vi "Unit Test Array of Classes.vi"() -> ()   [LabVIEW 2019, in "Sports Unit Tests.lvclass"]
uses:
  Sports Unit Tests.lvclass
  Classes/Shaquille ONeal/Shaquille O'Neal.lvclass
  C:/DSCE code/Serialization/blueserializationdemo/Test/Sports/Classes/Human/Human.lvclass
  C:/DSCE code/Serialization/blueserializationdemo/Test/Sports/Classes/Sports Player/Sports Player.lvclass
  Classes/Adam Sandler/Adam Sandler.lvclass
  C:/DSCE code/Serialization/blueserializationdemo/Test/Sports/Classes/Golf Player/Golf Player.lvclass
  Classes/Human/Human.lvclass/Human.ctl
  Classes/Sports Player/Sports Player.lvclass/Sports Player.ctl
  Classes/Golf Player/Golf Player.lvclass/Golf Player.ctl
  Classes/Adam Sandler/Adam Sandler.lvclass/Adam Sandler.ctl
  Classes/Shaquille ONeal/Shaquille O'Neal.lvclass/Shaquille O'Neal.ctl
  Classes/Sports Player/Sports Player.lvclass
  Classes/Human/Write Age (years).vi
  Classes/Human/Write alive_.vi
  Classes/Human/Write Height (ft).vi
  Classes/Human/Write Name.vi
  Classes/Sports Player/Write Earnings (dollars).vi
  Classes/Sports Player/Write Professional_.vi
  Classes/Sports Player/Write Sponsor.vi
  Classes/Golf Player/Write # holes in one.vi
  Classes/Golf Player/Write League.vi
  Classes/Golf Player/Write longest drive (ft).vi
  Classes/Adam Sandler/Write Movie Name.vi
  Classes/Adam Sandler/Write Private number.vi
  Classes/Adam Sandler/Write Secret phrase.vi
  Classes/Shaquille ONeal/Write #slam dunks.vi
  Classes/Shaquille ONeal/Write Nickname.vi
  <vilib>/Utility/error.llb/Clear Errors.vi
  <vilib>/addons/_JKI Toolkits/Caraya/classes/Test/Define Test.vi
  <vilib>/addons/_JKI Toolkits/Caraya/classes/Assert/Assert Equal Value_Variant.vi
  <vilib>/addons/_JKI Toolkits/Caraya/classes/Assert/Assert Not Error.vi
  <vilib>/addons/_JKI Toolkits/Caraya/classes/Assert/Assert.lvclass
  <userlib>/Blue Origin/BlueSerialization/BlueSerializer/BlueSerializer.lvclass
panel:
  out "Table":string[][](table)
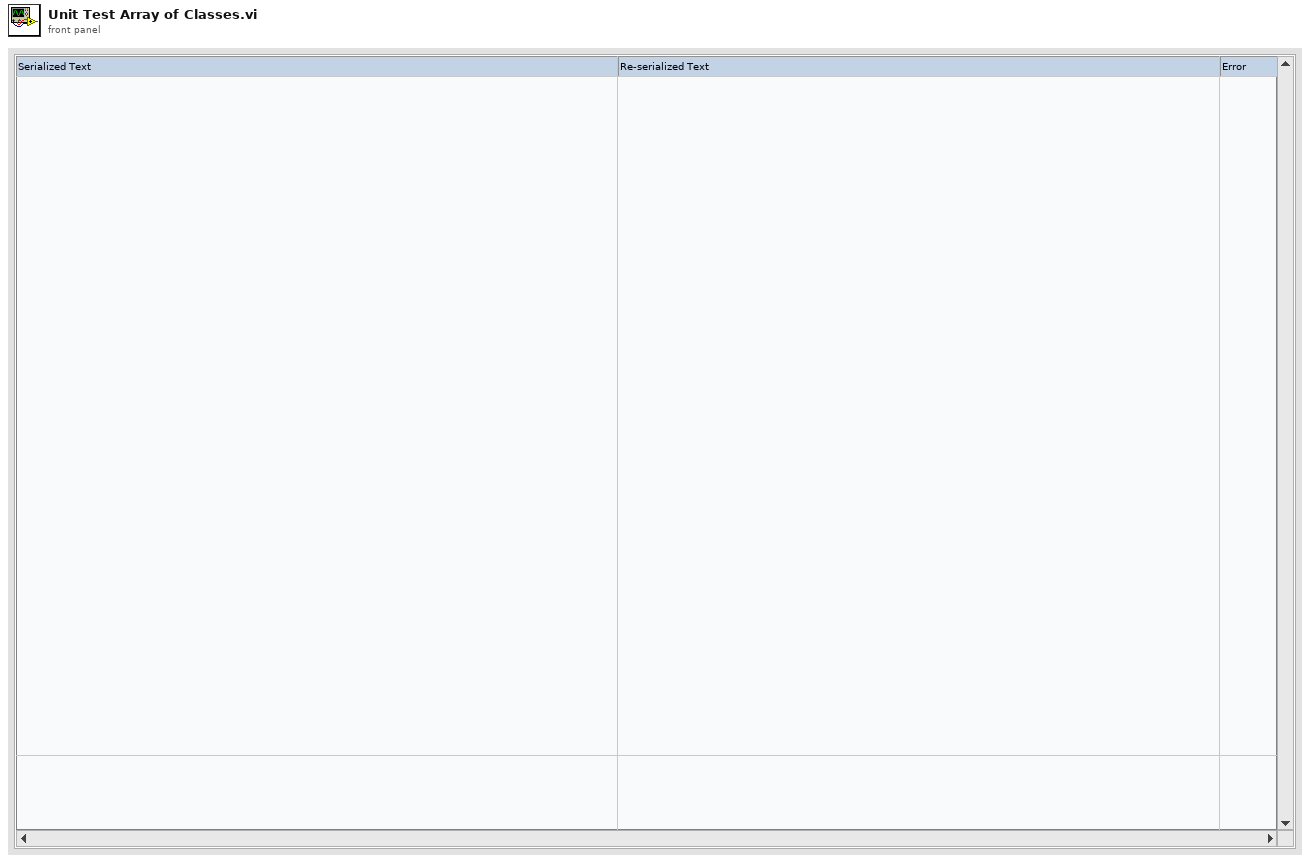
[diagram p1: front panel]
types:
  T1 = cluster{"Players":refnum<class "Sports Player.lvclass">[]}
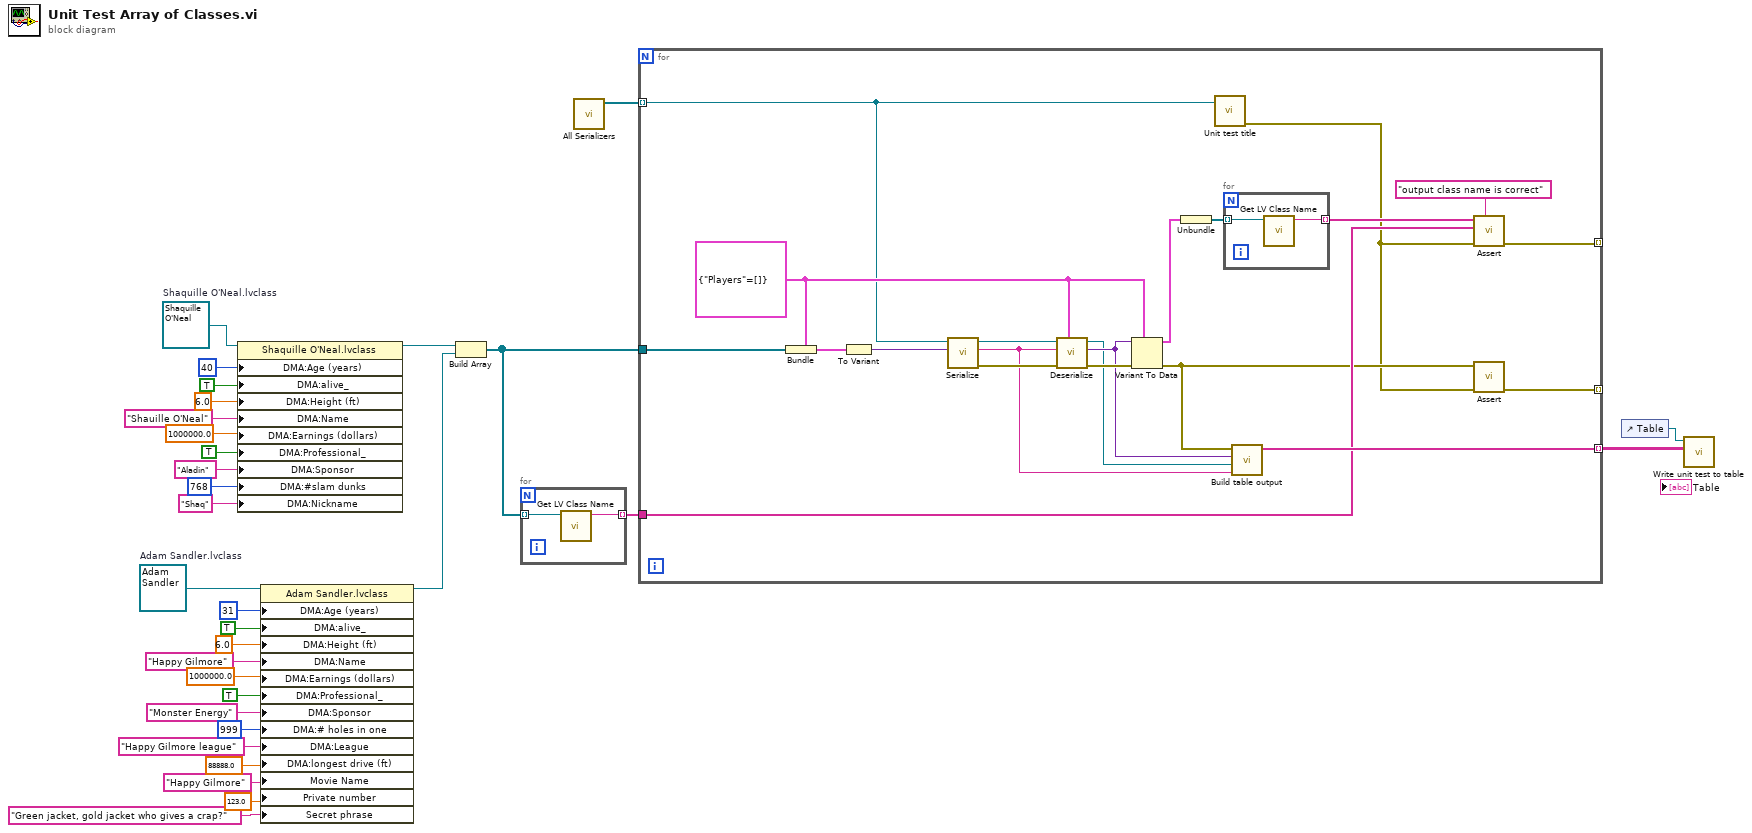
[diagram p0: block diagram]
diagram:
  w11 = refnum<class "Adam Sandler.lvclass"> refnum  # Adam Sandler.lvclass
  w21 = refnum<class "Shaquille O'Neal.lvclass"> refnum  # Shaquille O'Neal.lvclass
  n1 = property on="Property Node" class="Shaquille O'Neal.lvclass"(reference=w21, "DMA:Age (years)"=u16 40 ("Age (years)"), "DMA:alive_"=TRUE ("alive_"), "DMA:Height (ft)"=6.0 ("Height (ft)"), "DMA:Name"="Shauille O'Neal" ("Name"), "DMA:Earnings (dollars)"=1000000.0 ("Earnings (dollars)"), "DMA:Professional_"=TRUE ("Professional_"), "DMA:Sponsor"="Aladin" ("Sponsor"), "DMA:#slam dunks"=u64 768 ("#slam dunks"), "DMA:Nickname"="Shaq" ("Nickname")) -> (reference out=w4:refnum<class "Shaquille O'Neal.lvclass">)  [unwired: 1 in, 1 out]
  n2 = property on="Property Node" class="Adam Sandler.lvclass"(reference=w11, "DMA:Age (years)"=u16 31 ("Age (years)"), "DMA:alive_"=TRUE ("alive_"), "DMA:Height (ft)"=6.0 ("Height (ft)"), "DMA:Name"="Happy Gilmore" ("Name"), "DMA:Earnings (dollars)"=1000000.0 ("Earnings (dollars)"), "DMA:Professional_"=TRUE ("Professional_"), "DMA:Sponsor"="Monster Energy" ("Sponsor"), "DMA:# holes in one"=999 ("# holes in one"), "DMA:League"="Happy Gilmore league" ("League"), "DMA:longest drive (ft)"=88888.0 ("longest drive (ft)"), "Movie Name"="Happy Gilmore", "Private number"=123.0, "Secret phrase"="Green jacket, gold jacket who gives a crap?") -> (reference out=w3:refnum<class "Adam Sandler.lvclass">)  [unwired: 1 in, 1 out]
  n3 = Build Array(w4, w3) -> (w2:refnum<class "Sports Player.lvclass">[])
  n4 = for {
    tunnel: w2 -> [w33] mode=indexing
    tunnel: [w32] -> w1 mode=indexing
    n5 = call <vilib>:"Get LV Class Name.vi"("object"=w33) -> ("class name"=w32:string)  [unwired: 9 in, 1 out]
  }
  n6 = call "All Serializers.vi"() -> ("All serializers"=w30:refnum<class "BlueSerializer.lvclass">[])  [unwired: 11 in]
  n7 = for {
    tunnel: w30 -> [w34] mode=indexing
    tunnel: [w41] -> _ mode=indexing
    tunnel: [w50] -> _ mode=indexing
    tunnel: [w46] -> w29 mode=indexing
    tunnel: w2 -> [w40]
    tunnel: w1 -> [w44]
    w37 = T1 {"Players"=[]} ("cluster")
    n8 = Bundle(cluster=w37, "Players"=w40) -> (w39:T1)
    n9 = To Variant(anything=w39) -> (Variant=w38:variant)
    n10 = call <userlib>:"Serialize.vi"("Anything"=w38, "BlueSerializer in"=w34) -> ("error out"=w54:errorcluster, "Serialized Text"=w47:string, "BlueSerializer out"=w53:refnum<class "BlueSerializer.lvclass">)  [unwired: 7 in]
    n11 = call <userlib>:"Deserialize.vi"("Anything"=w37, "error in (no error)"=w54, "Serialized Text"=w47, "BlueSerializer in"=w53) -> ("error out"=w52:errorcluster, "Variant"=w49:variant, "BlueSerializer out"=w48:refnum<class "BlueSerializer.lvclass">)  [unwired: 5 in]
    n12 = Variant To Data(error in=w52, type=w37, Variant=w49) -> (data=w36:T1, error out=w43:errorcluster)
    n13 = Unbundle(w36) -> ("Players"=w35:refnum<class "Sports Player.lvclass">[])
    n14 = call "Unit test title.vi"("serializer"=w34) -> ("error out"=w42:errorcluster)  [unwired: 9 in, 1 out]
    n15 = for {
      tunnel: w35 -> [w56] mode=indexing
      tunnel: [w55] -> w45 mode=indexing
      n16 = call <vilib>:"Get LV Class Name.vi"("object"=w56) -> ("class name"=w55:string)  [unwired: 9 in, 1 out]
    }
    n17 = call "Build table output.vi"("serialized text"=w47, "BlueSerializer in"=w48, "deserialized variant"=w49, "variant to data error"=w43) -> ("table output"=w46:string[])  [unwired: 7 in]
    n18 = call-poly <vilib>:"Assert.vi"("Label"="output class name is correct", "error in (no error)"=w42, "Y"=w44, "X"=w45) -> ("error out"=w50:errorcluster)  [unwired: 7 in]
    n19 = call-poly <vilib>:"Assert.vi"("error in (no error)"=w42, "Not Error?"=w43) -> ("error out"=w41:errorcluster)  [unwired: 9 in]
  }
  n20 = control-ref of="Table"() -> (w31:refnum<vi>)
  n21 = call "Write unit test to table.vi"("Table"=w29, "Table ref in"=w31) -> ()  [unwired: 9 in, 1 out]
